vi "BotSpeak_GetVer.vi"(3 "Bot Settings":T1) -> (0 "version":string, 1 "Bot Settings out":T1)   [LabVIEW 2012]
doc: "Returns the version number of the device's VM"
uses:
  <userlib>/BotSpeak/VIs/Direct/BotSpeak_Control.ctl
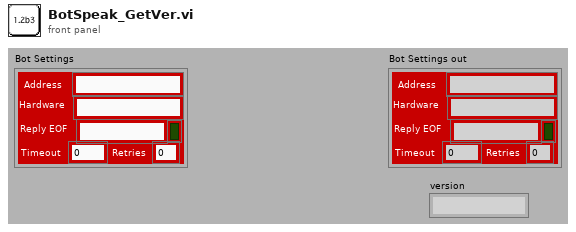
[diagram p1: front panel]
types:
  T1 = typedef "BotSpeak_Control.ctl" = cluster{"Address":string, "Reply EOF":string, "Hardware":string, "Retries":i8, "Timeout":i32, "Open?":bool}
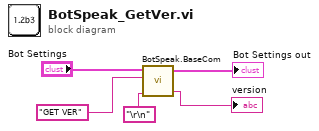
[diagram p0: block diagram]
diagram:
  n1 = call <userlib>:"BotSpeak.BaseCom.vi"("Termination"="\r\n", "command"="GET VER", "Bot Settings in"="Bot Settings") -> ("response"=→"version":string, "Bot Settings out"=→"Bot Settings out":T1)  [unwired: 2 in]
